vi "Stop Fast F Sweep.vi"(8 "error in (no error)":errorcluster, 11 "RUS settings":T1={"NI-DAQ lockin settings"={"Samples per sine wave"=0, "Sine waves per freq step"=0, "Output Representation"=enum."Real/Imaginary", "Low-pass filter"=enum."Butterworth", "Ranges and couplings "=[]}, "Fast swep settings"={"Update rate (Hz)"=250.0, "Start F, Hz"=200000.0, "Stop F"=1700000.0, "Number of points"=30000, "Amplitude"=2.1, "Init&amplitude"=TRUE, "IF"=1000.0, "Time constant"=0.1}, "Pre-sweep delay, s"=0.0, "Lockin mode"=enum."NI-DAQ", "SR Lockin"="GPIB0::10::INSTR", "DAQmx Device"="Dev3", "Clock Multiplier"=64, "Fast Sweep Data Out"={"DO clock task"="", "DO task"="", "Update clock task"="", "DAQ lockin task"="", "Pre-sweep counter task"=""}, "Lockin Range, V"=0.0, "F Array"=[], "Freq. update clock terminal"="", "DO Clock Rate (Hz)"=5000000.0, "ADC clock terminal"="/PFI4", "Pre-sweep counter terminal"="", "Samples per read"=10, "DO clock terminal"="", "Pre-sweep points"=0, "F points per write"=1000, "Total sweep time, s"=0.0, "Initial SYNTH phase"=0.0, "Record IF"=FALSE, "Save data settings"={"Save data"=TRUE, "Data Root Path"=path "", "File Prefix"="", "File Format"=enum."ASCII", "Save column names"=TRUE, "File Comments"="<Description of the current file>", "User/Prj"="<User Name/Project Description>"}, "Data file path"=path "", "New data user event"=refnum, "Stop user event"=refnum, "Number of channels"=1, "Auto-phase"=FALSE, "RP Transeiver"=refnum} {"Lockin Range, V" format="%#_6e"; "Fast swep settings"."IF" format="%#_6p"; "Fast swep settings"."Amplitude" min=0.0 max=2.5; "Fast swep settings"."Number of points" format="%.0p"; "Fast swep settings"."Stop F" format="%#_6p"; "Fast swep settings"."Start F, Hz" format="%#_6p"; "Fast swep settings"."Update rate (Hz)" format="%0.2f"; "NI-DAQ lockin settings"."Ranges and couplings"."Coupling" items=["default"=-1, "RSE"=10083, "NRSE"=10078, "Differential"=10106, "Pseudodifferential"=12529]}) -> (0 "error out":errorcluster)   [LabVIEW 2015]
uses:
  Controls/RUS settings.ctl
  NHMFL_Core/Libraries/Red Pitaya/RP Core/RP Transceiver/RP Transceiver.lvclass
  Controls/RUS NI-DAQ Lockin Settings.ctl
  Controls/Sweep settings.ctl
  Controls/Lockin mode.ctl
  NHMFL_Core/Libraries/File/Controls/Save data settings.ctl
  NHMFL_Core/Libraries/File/Controls/File formats.ctl
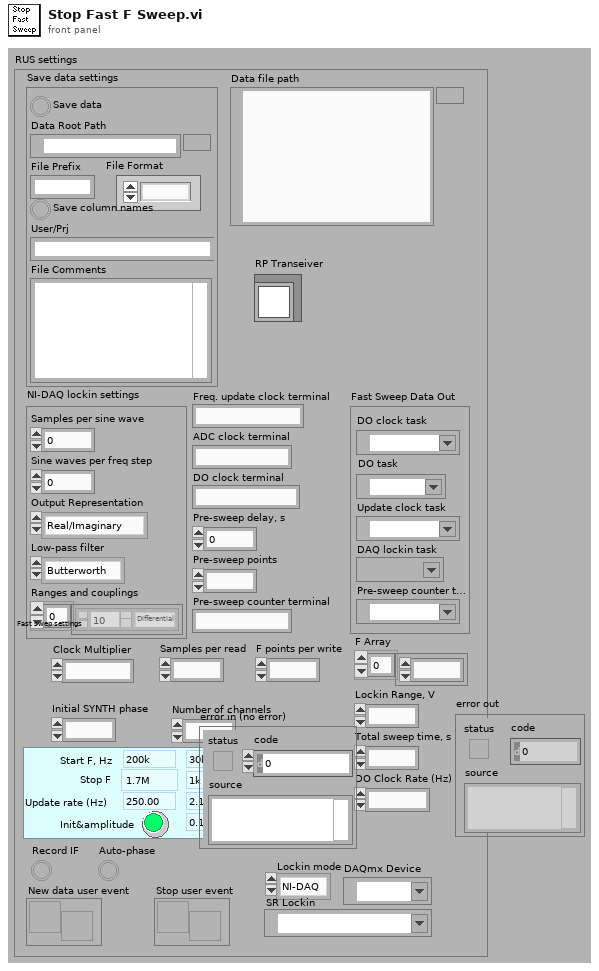
[diagram p1: front panel]
types:
  T1 = typedef "RUS settings.ctl" = cluster{"NI-DAQ lockin settings":T2, "Fast swep settings":T3, "Pre-sweep delay, s":dbl, "Lockin mode":T4, "SR Lockin":refnum<visa-resource-name>, "DAQmx Device":tag, "Clock Multiplier":i32, "Fast Sweep Data Out":cluster{"DO clock task":refnum<k21>, "DO task":refnum<k21>, "Update clock task":refnum<k21>, "DAQ lockin task":refnum<k21>, "Pre-sweep counter task":refnum<k21>}, "Lockin Range, V":sgl, "F Array":dbl[], "Freq. update clock terminal":string, "DO Clock Rate (Hz)":dbl, "ADC clock terminal":string, "Pre-sweep counter terminal":string, "Samples per read":i32, "DO clock terminal":string, "Pre-sweep points":i32, "F points per write":i32, "Total sweep time, s":dbl, "Initial SYNTH phase":dbl, "Record IF":bool, "Save data settings":T5, "Data file path":path, "New data user event":refnum<user-event>, "Stop user event":refnum<user-event>, "Number of channels":i32, "Auto-phase":bool, "RP Transeiver":refnum<class "RP Transceiver.lvclass">}
  T2 = typedef "RUS NI-DAQ Lockin Settings.ctl" = cluster{"Samples per sine wave":i32, "Sine waves per freq step":i32, "Output Representation":enum16{"Real/Imaginary", "Polar"}, "Low-pass filter":enum16{"No filtering", "Butterworth", "Bessel"}, "Ranges and couplings ":cluster{"Range":dbl, "Coupling":i32}[]}
  T3 = typedef "Sweep settings.ctl" = cluster{"Update rate (Hz)":dbl, "Start F, Hz":dbl, "Stop F":dbl, "Number of points":i32, "Amplitude":dbl, "Init&amplitude":bool, "IF":dbl, "Time constant":dbl}
  T4 = typedef "Lockin mode.ctl" = enum16{"SRS", "NI-DAQ", "Pitaya"}
  T5 = typedef "Save data settings.ctl" = cluster{"Save data":bool, "Data Root Path":path, "File Prefix":string, "File Format":T6, "Save column names":bool, "File Comments":string, "User/Prj":string}
  T6 = typedef "File formats.ctl" = enum16{"TDMS", "ASCII", "BINARY"}
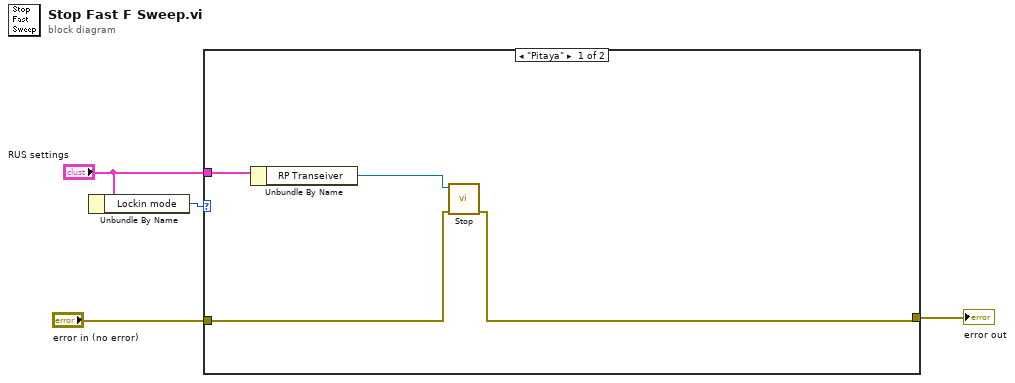
[diagram p0: block diagram]
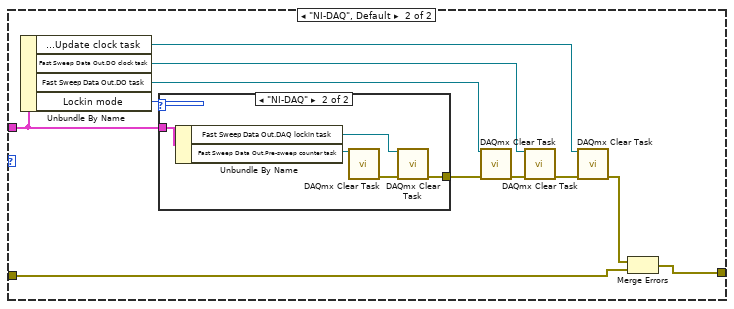
[diagram p2: hidden frame]
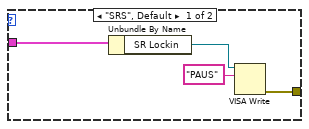
[diagram p3: hidden frame]
diagram:
  n1 = Unbundle By Name("RUS settings") -> ("Lockin mode"=w1:T4)
  n2 = case shown="\"Pitaya\"" w1 {
    tunnel: "error in (no error)" -> [w6 w13]
    tunnel: [w5 w12] -> w3
    tunnel: "RUS settings" -> [w8 w9]
    frame "Pitaya" {
      n3 = Unbundle By Name(w8) -> ("RP Transeiver"=w7:refnum<class "RP Transceiver.lvclass">)
      n4 = call-dynamic "Stop.vi"("error in (no error)"=w6, "RP Transceiver in"=w7) -> ("error out"=w5:errorcluster)  [unwired: 8 in, 1 out]
    }
    frame "NI-DAQ", Default {
      n5 = Unbundle By Name(w9) -> ("Fast Sweep Data Out.Update clock task"=w15:refnum<k21>, "Fast Sweep Data Out.DO clock task"=w16:refnum<k21>, "Fast Sweep Data Out.DO task"=w17:refnum<k21>, "Lockin mode"=w11:T4)
      n6 = case shown="\"NI-DAQ\"" w11 {
        tunnel: [w23 w27] -> w14
        tunnel: w9 -> [w21 w26]
        frame "SRS", Default {
          n7 = Unbundle By Name(w21) -> ("SR Lockin"=w20:refnum<visa-resource-name>)
          n8 = VISA Write(VISA resource name=w20, write buffer="PAUS") -> (error out=w23:errorcluster)  [unwired: 1 in, 2 out]
        }
        frame "NI-DAQ" {
          n9 = Unbundle By Name(w26) -> ("Fast Sweep Data Out.DAQ lockin task"=w25:refnum<k21>, "Fast Sweep Data Out.Pre-sweep counter task"=w24:refnum<k21>)
          n10 = call <vilib>:"DAQmx Clear Task.vi"("task in"=w24) -> ("error out"=w28:errorcluster)  [unwired: 1 in, 13 out]
          n11 = call <vilib>:"DAQmx Clear Task.vi"("task in"=w25, "error in"=w28) -> ("error out"=w27:errorcluster)  [unwired: 13 out]
        }
      }
      n12 = call <vilib>:"DAQmx Clear Task.vi"("task in"=w17, "error in"=w14) -> ("error out"=w19:errorcluster)  [unwired: 13 out]
      n13 = call <vilib>:"DAQmx Clear Task.vi"("task in"=w16, "error in"=w19) -> ("error out"=w18:errorcluster)  [unwired: 13 out]
      n14 = call <vilib>:"DAQmx Clear Task.vi"("task in"=w15, "error in"=w18) -> ("error out"=w10:errorcluster)  [unwired: 13 out]
      n15 = Merge Errors(w10, w13) -> (w12:errorcluster)
    }
  }
  "error out" <- w3
